vi "Generate Histogram.vi"(8 "error in (no error)":errorcluster, 10 "Interval Scaling":i32=10 min=1, 11 "Performance Analyzer In":T1) -> (0 "error out":errorcluster, 2 "Histogram":cluster{dbl, dbl}[](graph), 3 "Performance Analyzer Out":T1)   [LabVIEW 2020]
uses:
  Data Cluster.ctl
  Helper Classes/Test Finder/Test Finder.lvclass
  <vilib>/Analysis/NI_AALBase.lvlib
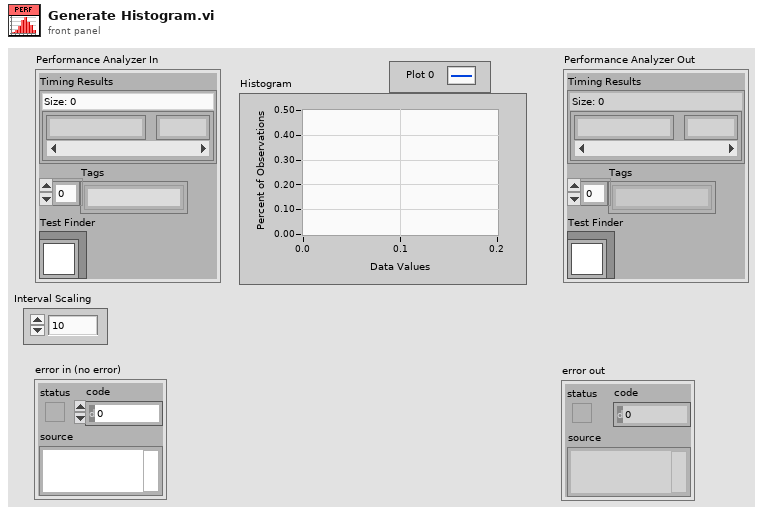
[diagram p1: front panel]
types:
  T1 = typedef "Data Cluster.ctl" = cluster{"Timing Results":map{string, dbl}, "Tags":string[], "Test Finder":refnum<class "Test Finder.lvclass">}
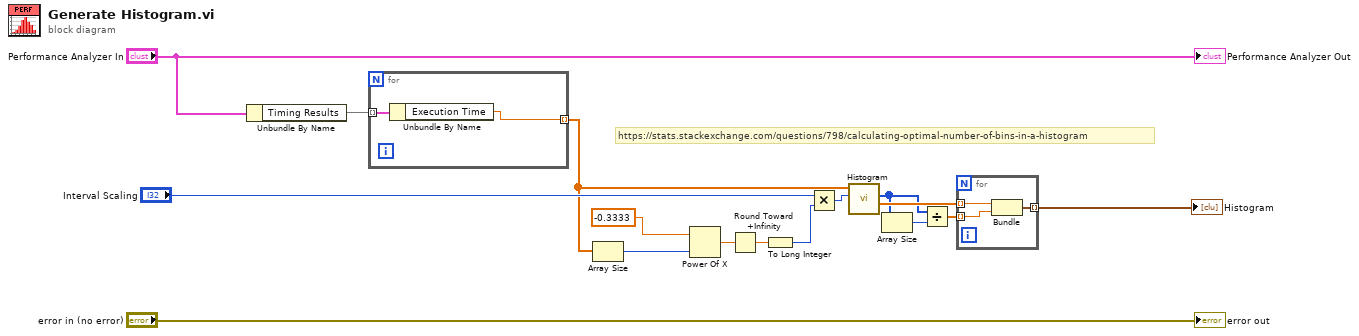
[diagram p0: block diagram]
diagram:
  # "https://stats.stackexchange.com/questions/798/calculating-optimal-number-of-bins-in-a-histogram"
  n1 = Unbundle By Name("Performance Analyzer In") -> ("Timing Results"=w8:map{string, dbl})
  n2 = for {
    tunnel: w8 -> [w18] mode=indexing
    tunnel: [w17] -> w7 mode=indexing
    n3 = Unbundle By Name(w18) -> ("Execution Time"=w17:dbl)
  }
  n4 = Array Size(array=w7) -> (size(s)=w6:i32)
  n5 = Power Of X(1:w6, 2:-0.3333 ("y")) -> (0:w4:dbl)
  n6 = Round Toward +Infinity(x=w4) -> (ceil(x): smallest int >= x=w3:dbl)
  n7 = To Long Integer(number=w3) -> (32bit integer=w2:i32)
  n8 = Multiply(x="Interval Scaling", y=w2) -> (x*y=w5:i32)
  n9 = call <vilib>:"Histogram.vi"("intervals"=w5, "X"=w7) -> ("X Values"=w13:dbl[], "Histogram: h(x)"=w10:i32[])  [unwired: 6 in, 2 out]
  n10 = Array Size(array=w10) -> (size(s)=w12:i32)
  n11 = Divide(x=w10, y=w12) -> (x/y=w11:dbl[])
  n12 = for {
    tunnel: w11 -> [w20] mode=indexing
    tunnel: [w21] -> w14 mode=indexing
    tunnel: w13 -> [w19] mode=indexing
    n13 = Bundle(w19, w20) -> (w21:cluster{dbl, dbl})  [unwired: 1 in]
  }
  "Histogram" <- w14
  "error out" <- "error in (no error)"
  "Performance Analyzer Out" <- "Performance Analyzer In"
